vi "Reserve Callback.vi"(8 "error in (no error)":errorcluster, 10 "session reservation":refnum<class "Session Reservation.lvclass">, 11 "reservation observer in":refnum<class "Reservation Observer.lvclass">) -> (0 "error out":errorcluster, 3 "reservation observer out":refnum<class "Reservation Observer.lvclass">)   [LabVIEW 2020, in "MeasurementLink Measurement Server.lvlib" / "Reservation Observer.lvclass"]
uses:
  Reservation Observer.lvclass
  MeasurementLink Session Management/Session Reservation/Session Reservation.lvclass
  Reservation Observer.lvclass/Reservation Observer.ctl
  Classes/MeasurementContext/MeasurementContext.lvclass
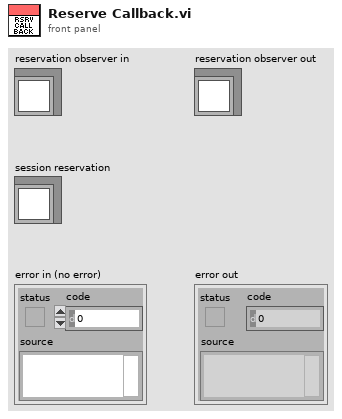
[diagram p1: front panel]
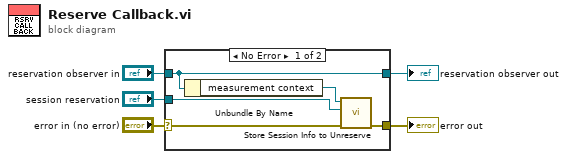
[diagram p0: block diagram]
diagram:
  n1 = case shown="No Error" "error in (no error)" {
    selector: "error in (no error)" -> [w8 w12]
    tunnel: "reservation observer in" -> [w7 w11]
    tunnel: [w9 w12] -> w4
    tunnel: [w7 w11] -> w2
    tunnel: "session reservation" -> [w6 _]
    frame No Error {
      n2 = Unbundle By Name(w7) -> ("measurement context"=w10:refnum<class "MeasurementContext.lvclass">)
      n3 = call "Store Session Info to Unreserve.vi"("error in"=w8, "session reservation"=w6, "measurement context in"=w10) -> ("error out"=w9:errorcluster)  [unwired: 7 in, 1 out]
    }
    frame Error {
    }
  }
  "error out" <- w4
  "reservation observer out" <- w2
